vi "c ctre phoenixpro Request Control BMS Manual Isolator.vi"(6 "Enable":bool, 7 "cancelOtherRequests":bool, 8 "error in (no error)":errorcluster, 9 "updateTime":dbl, 10 "ecuEncoding":u32, 11 "canbus":string) -> (0 "error out":errorcluster, 3 "function return":i32)   [LabVIEW 2020, in "CTRE_PhoenixTools.lvlib"]
doc: "CTREXPORT int c_ctre_phoenixpro_RequestControlBMSManualIsolator(const char *canbus, uint32_t ecuEncoding, double updateTime, bool cancelOtherRequests, bool Enable);"
uses:
  CTRE_PhoenixTools.lvlib
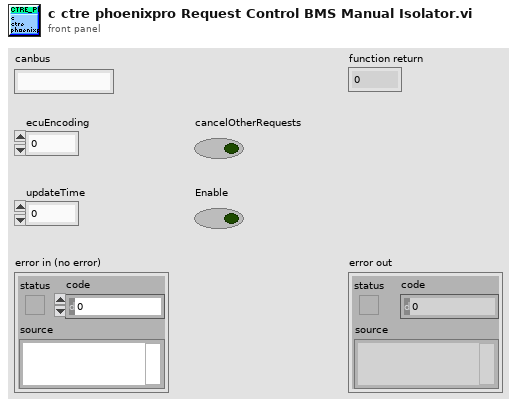
[diagram p1: front panel]
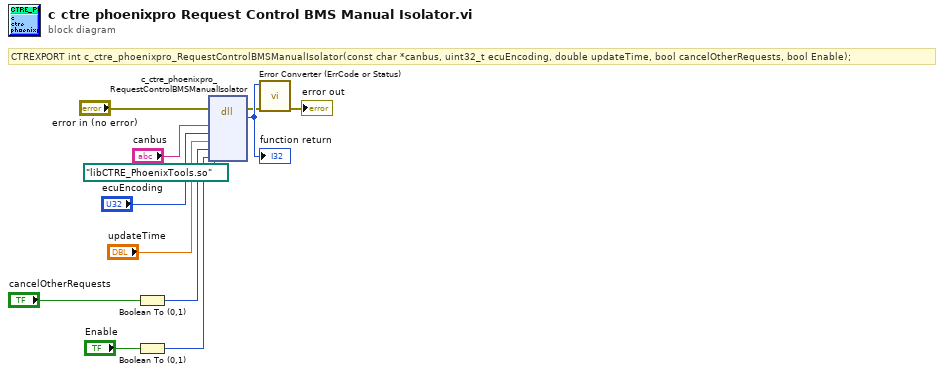
[diagram p0: block diagram]
diagram:
  # "CTREXPORT int c_ctre_phoenixpro_RequestControlBMSManualIsolator(const char *canbus, uint32_t ecuEncoding, double updateTime, bool cancelOtherRequests, bool Enable);"
  n1 = Boolean To (0,1)(Boolean="cancelOtherRequests") -> (0, 1=w7:i16)
  n2 = Boolean To (0,1)(Boolean="Enable") -> (0, 1=w5:i16)
  n3 = dll-call lib="?" fn="c_ctre_phoenixpro_RequestControlBMSManualIsolator"(path in=path "libCTRE_PhoenixTools.so", error in="error in (no error)", "canbus"="canbus", "ecuEncoding"="ecuEncoding", "updateTime"="updateTime", "cancelOtherRequests"=w7, "Enable"=w5) -> (error out=w3:errorcluster, "return type"=w12:i32)  [unwired: 6 in, 1 out]
  "function return" <- w12
  n4 = call "Error Converter (ErrCode or Status).vi"("error in (no error)"=w3, "error code"=w12) -> ("error out"=→"error out":errorcluster)  [unwired: 9 in]
